vi "Read Encoders.vi"(8 "error in (no error)":errorcluster, 9 "DUT1":bool, 10 "No samples":u32=1000, 11 "task in":i32) -> (0 "error out":errorcluster, 1 "CW/CCW":bool, 2 "Stopped":bool, 3 "task out":i32)   [LabVIEW 2023]
uses:
  <userlib>/DAQNavi Polymorphic VI/read/DAQNavi Read (Digital 1D Wfm NChan NSamp).vi
panel:
  out "Digital Waveform Graph":digitalwaveform[](graph)
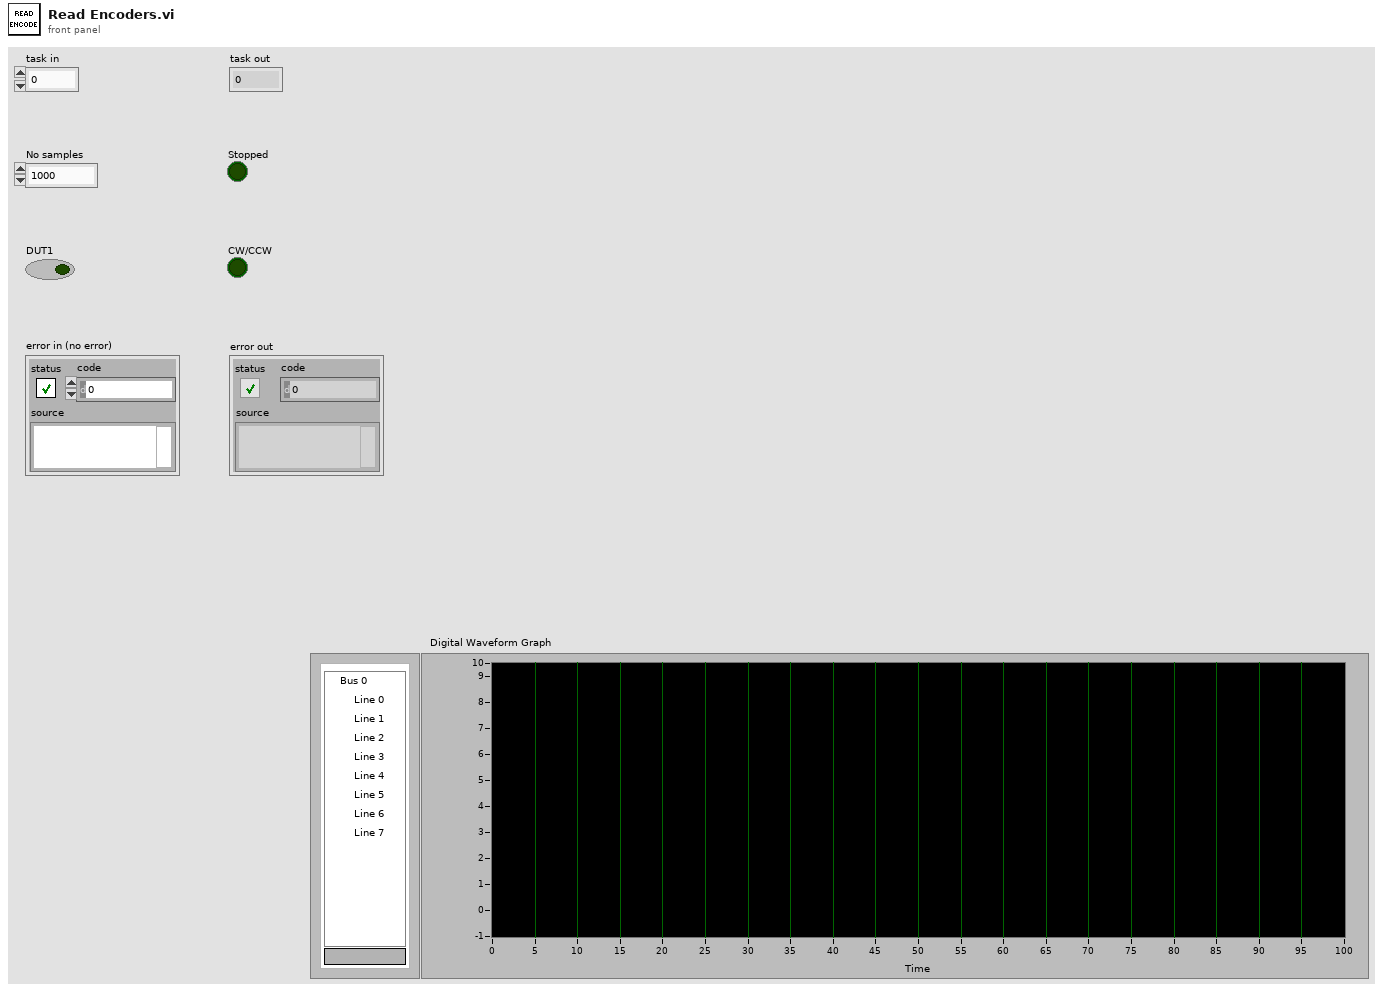
[diagram p1: front panel]
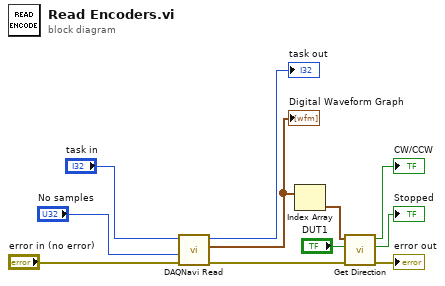
[diagram p0: block diagram]
diagram:
  n1 = call-poly <userlib>:"DAQNavi Read.vi"("error in (no error)"="error in (no error)", "number of samples per channel to read"="No samples", "task in"="task in") -> ("error out"=w7:errorcluster, "data"=w2:digitalwaveform[], "task out"=→"task out":i32)  [unwired: 1 in, 5 out]
  "Digital Waveform Graph" <- w2
  n2 = Index Array(array=w2) -> (element=w1:digitalwaveform)  [unwired: 1 in]
  n3 = call "Get Direction.vi"("error in (no error)"=w7, "DUT1"="DUT1", "Measured signal"=w1) -> ("error out"=→"error out":errorcluster, "Stopped"=→"Stopped":bool, "CW/CCW"=→"CW/CCW":bool)  [unwired: 6 in]
